vi "Main Analysis-Labial.vi"(0 "selected path":path, 5 "VI reference":refnum<vi>, 11 "Error In":errorcluster) -> (3 "error?":bool, 4 "File Path Indicator":path, 6 "Pressure Array":dbl[](array[numeric]), 8 "SPL Array":dbl[](array[numeric]), 10 "Mean Flow (Overall)":dbl format="%0.3f", 14 "F0 Array":dbl[](array[numeric]), 15 "Error Out":errorcluster)   [LabVIEW 2018, in "MainVIs.lvlib"]
uses:
  MainVIs.lvlib
  AnalysisSupport.lvlib
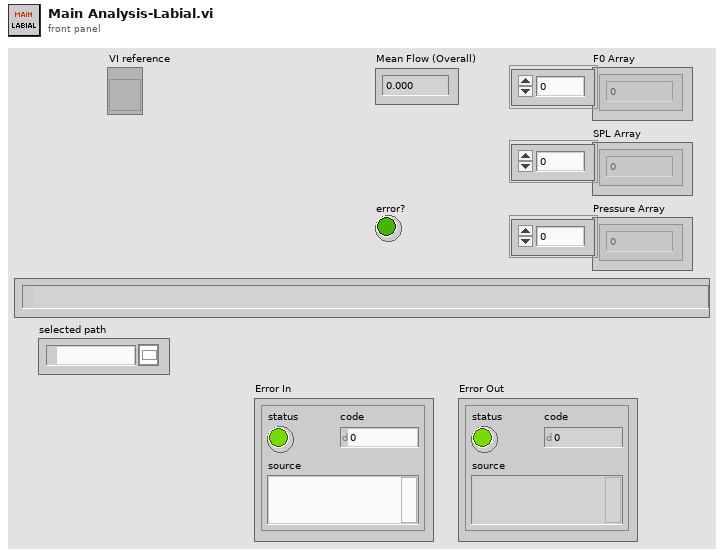
[diagram p1: front panel]
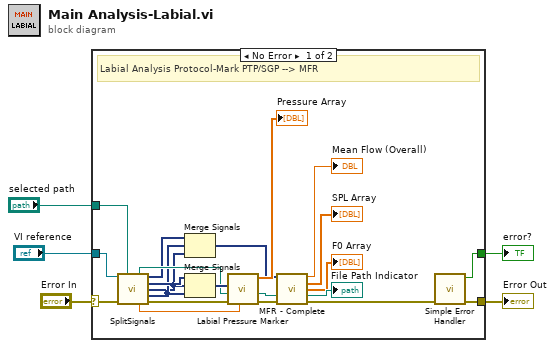
[diagram p0: block diagram]
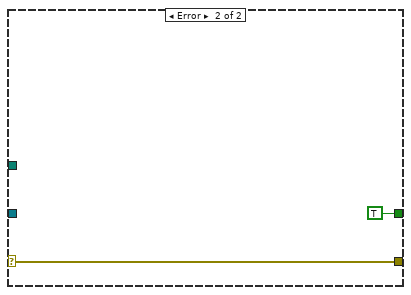
[diagram p2: hidden frame]
diagram:
  n1 = case shown="No Error" "Error In" {
    selector: "Error In" -> [w27 w29]
    tunnel: "selected path" -> [w26 _]
    tunnel: [w24 w29] -> w3
    tunnel: [w23 TRUE ("error?")] -> w2
    tunnel: "VI reference" -> [w8 _]
    frame No Error {
      # "Labial Analysis Protocol-Mark PTP/SGP --> MFR"
      n2 = call "SplitSignals.vi"("VI reference"=w8, "Filename"=w26, "Error In"=w27) -> ("Filename Out"=w19:path, "Flow"=w13:dynamicdata, "Pressure"=w25:dynamicdata, "Audio"=w6:dynamicdata, "SPL"=w12:dynamicdata, "Upper SPL"=w9:dbl, "Error Out"=w21:errorcluster)  [unwired: 5 in, 1 out]
      n3 = Merge Signals(w13, w12, w6) -> (w11:dynamicdata)
      n4 = Merge Signals(w25, w6, w12) -> (w22:dynamicdata)
      n5 = call "Labial Pressure Marker.vi"("Upper SPL"=w9, "Error In"=w21, "File Path"=w19, "Pressure/Audio"=w22) -> ("Error Out"=w16:errorcluster, "File Path Indicator"=w15:path, "Pressure Array"=→"Pressure Array":dbl[])  [unwired: 5 in]
      n6 = call "MFR - Complete.vi"("Flow, SPL & Audio"=w11, "File Name In"=w15, "Error In"=w16) -> ("Mean Flow (Overall)"=→"Mean Flow (Overall)":dbl, "SPL Array"=→"SPL Array":dbl[], "F0 Array"=→"F0 Array":dbl[], "File Name"=→"File Path Indicator":path, "Error Out"=w17:errorcluster)  [unwired: 8 in]
      n7 = call <vilib>:"Simple Error Handler.vi"("error in (no error)"=w17) -> ("error?"=w23:bool, "error out"=w24:errorcluster)  [unwired: 4 in, 3 out]
    }
    frame Error {
    }
  }
  "Error Out" <- w3
  "error?" <- w2
